vi "ZCAN_StartCAN.vi"(8 "error in (no error)":errorcluster, 11 "can_index_handle":u32) -> (0 "error out":errorcluster, 3 "can_index_handle(out)":u32)   [LabVIEW 2020, in "zlgcan.lvlib"]
uses:
  zlgcan.lvlib
  bin/zlgcan_wrap.dll
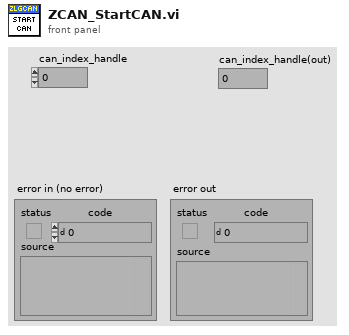
[diagram p1: front panel]
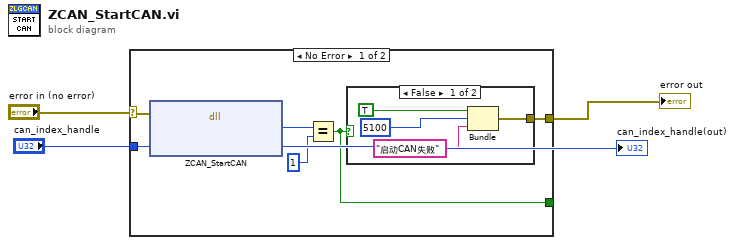
[diagram p0: block diagram]
diagram:
  n1 = case shown="No Error" "error in (no error)" {
    selector: "error in (no error)" -> [w7 w14]
    tunnel: [w5 w14] -> w1
    tunnel: "can_index_handle" -> [w6 _]
    tunnel: [w4 _] -> _
    frame No Error {
      n2 = dll-call lib="D:/Git/ZLG_USBCANFD/bin/zlgcan_wrap.dll" fn="ZCAN_StartCAN"(error in=w7, "can_handle"=w6) -> ("return"=w9:u32)  [unwired: 3 in, 2 out]
      n3 = Equal?(x=w9, y=1) -> (x = y?=w4:bool)
      n4 = case shown="False" w4 {
        tunnel: [w10 _] -> w5
        frame False {
          n5 = Bundle("status"=TRUE, "code"=5100, "消息"="启动CAN失败") -> (w10:cluster{"status":bool, "code":i32, "消息":string})  [unwired: 1 in]
        }
        frame True {
        }
      }
    }
    frame Error {
    }
  }
  "error out" <- w1
  "can_index_handle(out)" <- "can_index_handle"
